vi "Excel Workbook Properties.vi"(0 "report in":refnum<class "NI_report.lvclass">, 1 "title (\"\")":string, 5 "subject (\"\")":string, 7 "author (\"\")":string, 9 "comments (\"\")":string, 11 "error in (no error)":errorcluster) -> (4 "report out":refnum<class "NI_report.lvclass">, 8 "worksheets count":i32, 10 "current worksheet name":string, 15 "error out":errorcluster)   [LabVIEW 2017, in "NI_ReportGenerationToolkit.lvlib"]
doc: "Sets the properties of the current workbook, such as the author, title, and subject. You also can use this VI to return the number of worksheets in the current workbook."
uses:
  <vilib>/addons/_office/NI_ReportGenerationToolkit.lvlib
  <vilib>/Utility/NIReport.llb/NI_report.lvclass
  <vilib>/Utility/NIReport.llb/Excel/NI_Excel.lvclass
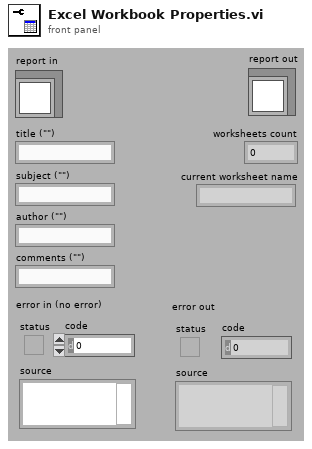
[diagram p1: front panel]
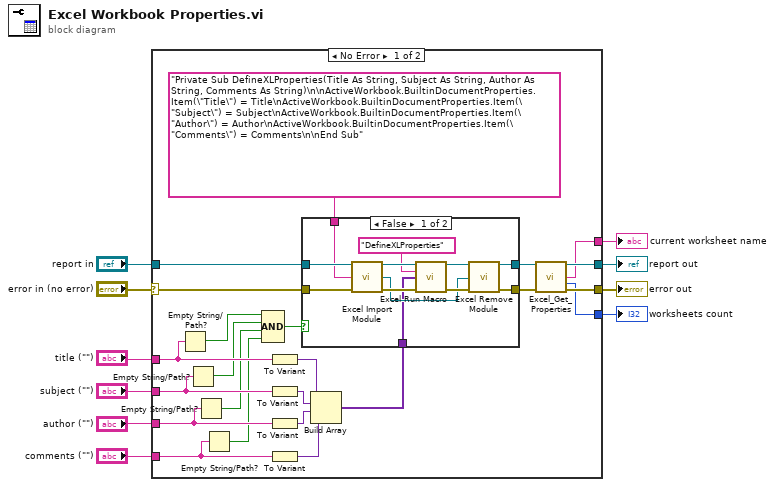
[diagram p0: block diagram]
diagram:
  n1 = case shown="No Error" "error in (no error)" {
    selector: "error in (no error)" -> [w11 w48]
    tunnel: "report in" -> [w32 w49]
    tunnel: "title (\"\")" -> [w27 _]
    tunnel: "subject (\"\")" -> [w26 _]
    tunnel: "author (\"\")" -> [w25 _]
    tunnel: "comments (\"\")" -> [w24 _]
    tunnel: [w16 w48] -> w5
    tunnel: [w15 w49] -> w4
    tunnel: [w13 _] -> w3
    tunnel: [w12 _] -> w2
    frame No Error {
      n2 = Empty String/Path?(string/path=w27) -> (empty?=w23:bool)
      n3 = Empty String/Path?(string/path=w26) -> (empty?=w22:bool)
      n4 = Empty String/Path?(string/path=w25) -> (empty?=w21:bool)
      n5 = Empty String/Path?(string/path=w24) -> (empty?=w20:bool)
      n6 = Compound Arithmetic op=AND(w23, w22, w21, w20) -> (w19:bool)
      n7 = To Variant(anything=w27) -> (Variant=w31:variant)
      n8 = To Variant(anything=w26) -> (Variant=w29:variant)
      n9 = To Variant(anything=w25) -> (Variant=w28:variant)
      n10 = To Variant(anything=w24) -> (Variant=w30:variant)
      n11 = Build Array(w31, w29, w28, w30) -> (w33:variant[])
      n12 = case shown="False" w19 {
        tunnel: w33 -> [w39 _]
        tunnel: w32 -> [w38 w47]
        tunnel: w11 -> [w37 w46]
        tunnel: [w36 w47] -> w17
        tunnel: [w35 w46] -> w18
        tunnel: "Private Sub DefineXLProperties(Title As String, Subject As String, Author As String, Comments As String)\n\nActiveWorkbook.BuiltinDocumentProperties.Item(\"Title\") = Title\nActiveWorkbook.BuiltinDocumentProperties.Item(\"Subject\") = Subject\nActiveWorkbook.BuiltinDocumentProperties.Item(\"Author\") = Author\nActiveWorkbook.BuiltinDocumentProperties.Item(\"Comments\") = Comments\n\nEnd Sub" -> [w34 _]
        frame False {
          n13 = call <vilib>:"Excel Import Module.vi"("report in"=w38, "module code (\"\")"=w34, "error in (no error)"=w37) -> ("report out"=w43:refnum<class "NI_report.lvclass">, "module reference"=w41:refnum<k7>, "error out"=w45:errorcluster)  [unwired: 1 in, 9 out]
          n14 = call <vilib>:"Excel Run Macro.vi"("report in"=w43, "macro name"="DefineXLProperties", "parameters"=w39, "error in (no error)"=w45) -> ("report out"=w42:refnum<class "NI_report.lvclass">, "error out"=w44:errorcluster)  [unwired: 10 out]
          n15 = call <vilib>:"Excel Remove Module.vi"("report in"=w42, "module reference"=w41, "error in (no error)"=w44) -> ("report out"=w36:refnum<class "NI_report.lvclass">, "error out"=w35:errorcluster)  [unwired: 11 out]
        }
        frame True {
        }
      }
      n16 = call <vilib>:"Excel_Get_Properties.vi"("report in"=w17, "error in (no error)"=w18) -> ("report out"=w15:refnum<class "NI_report.lvclass">, "current worksheet name"=w12:string, "worksheets count"=w13:i32, "error out"=w16:errorcluster)  [unwired: 10 out]
    }
    frame Error {
    }
  }
  "report out" <- w4
  "error out" <- w5
  "worksheets count" <- w3
  "current worksheet name" <- w2
